vi "FP_Pane Set Origin.vi"(8 "Error":errorcluster, 9 "Border Spacing":i16, 10 "FP Position":T1, 11 "Pane":refnum<vi>) -> (0 "Error Out":errorcluster, 3 "Pane In Out":refnum<vi>)   [LabVIEW 2024]
uses:
  <vilib>/Utility/miscctls.llb/LVPositionTypeDef.ctl
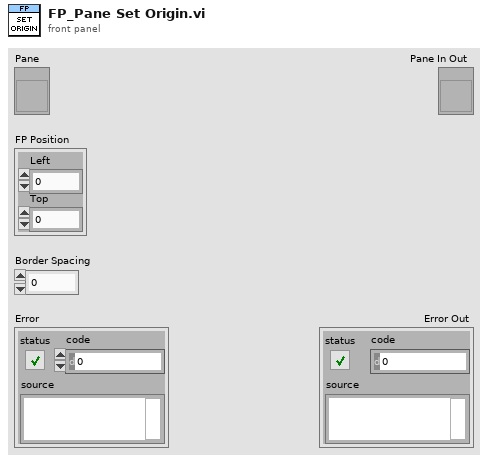
[diagram p1: front panel]
types:
  T1 = typedef "LVPositionTypeDef.ctl" = cluster{"Left":i32, "Top":i32}
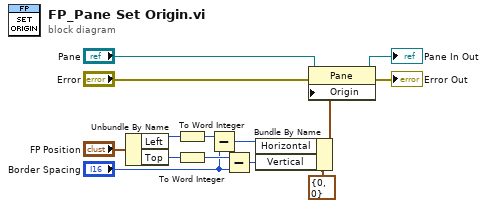
[diagram p0: block diagram]
diagram:
  n1 = Unbundle By Name("FP Position") -> ("Left"=w13:i32, "Top"=w14:i32)
  n2 = To Word Integer(number=w13) -> (16bit integer=w4:i16)
  n3 = To Word Integer(number=w14) -> (16bit integer=w3:i16)
  n4 = Subtract(x=w4, y="Border Spacing") -> (x-y=w6:i16)
  n5 = Subtract(x=w3, y="Border Spacing") -> (x-y=w7:i16)
  n6 = Bundle By Name(cluster=cluster{"Horizontal":i16, "Vertical":i16} {"Horizontal"=0, "Vertical"=0} ("Front Panel Window:Origin"), "Horizontal"=w6, "Vertical"=w7) -> (w9:cluster{"Horizontal":i16, "Vertical":i16})
  n7 = property on="Property Node" class="Pane"(reference="Pane", error in="Error", "Origin"=w9) -> (reference out=→"Pane In Out":refnum<vi>, error out=→"Error Out":errorcluster)
